vi "ROIAroundGaussian.vi"(9 "Resolution":cluster{"X Step":u16, "Y Step":u16}={"X Step"=1280, "Y Step"=1024}, 10 "Rangefactor (multiple w)":dbl=3.0, 11 "Fit Pixel":dbl[](array[numeric])) -> (0 "Subsampling":i32(ring)=16 items=["1"=1, "2"=2, "4"=4, "8"=8, "16"=16], 1 "ROI Offset":i32[](array[numeric]), 2 "Rectangle":T2 {"Rotation" min=-90.0 max=90.0 step=1.0 format="%.2f"; "Left" scale=0.0..1024.0; "Right" scale=0.0..1024.0}, 3 "ROI":T1, 4 "ROI Width":dbl, 5 "Rectangle (Array)":i32[](array[numeric]))   [LabVIEW 2015]
panel:
  # "x"
  # "pixels"
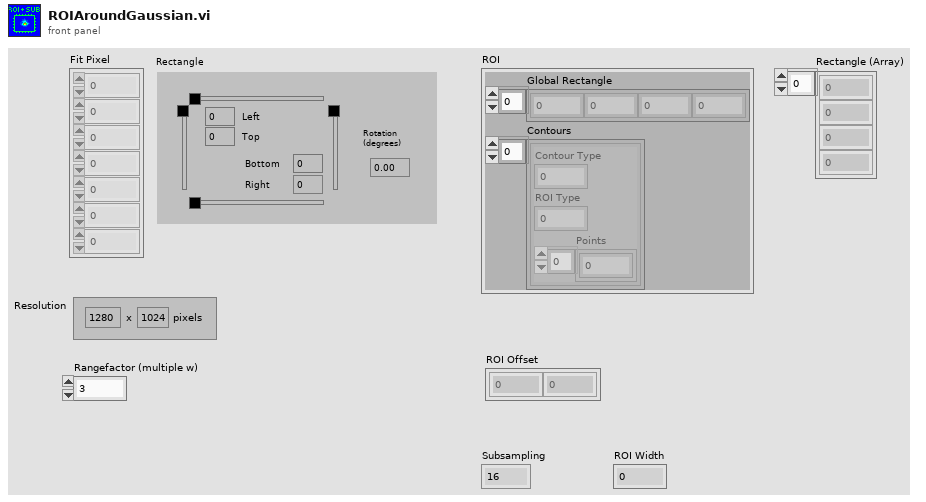
[diagram p1: front panel]
types:
  T1 = cluster{"Global Rectangle":i32[], "Contours":cluster{"Contour Type":u32, "ROI Type":u32, "Points":i32[]}[]}
  T2 = typedef "IMAQ Rectangle" = cluster{"Left":i32, "Top":i32, "Right":i32, "Bottom":i32, "Rotation":dbl}
  T3 = typedef "ROI Descriptor" = cluster{"Global Rectangle":i32[], "Contours":cluster{"ID":enum32{"External", "Internal"}, "Type":u32, "Coordinates":i32[]}[]}
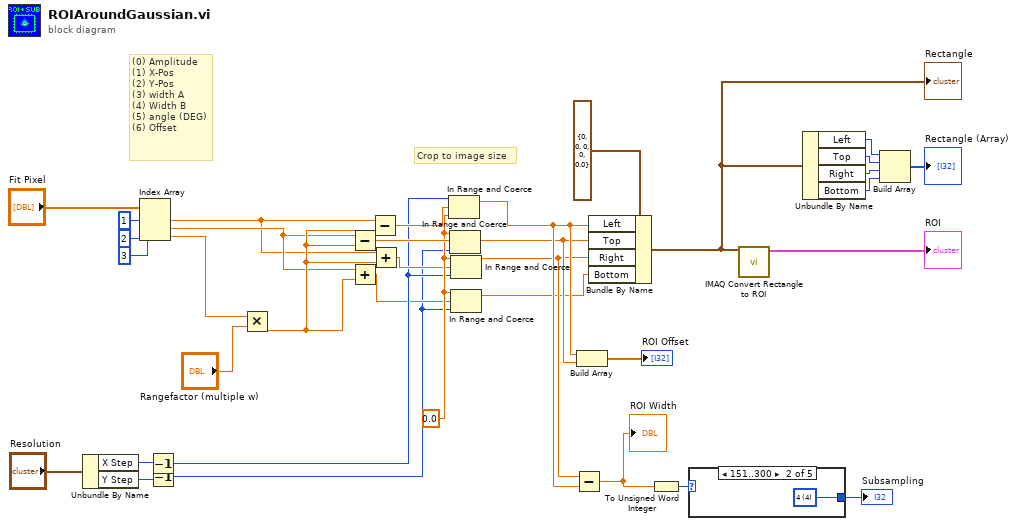
[diagram p0: block diagram]
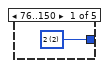
[diagram p2: hidden frame]
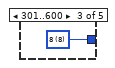
[diagram p3: hidden frame]
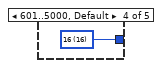
[diagram p4: hidden frame]
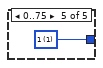
[diagram p5: hidden frame]
diagram:
  w14 = 0.0 ("lower limit")
  # "Crop to image size"
  # "(0) Amplitude\n(1) X-Pos\n(2) Y-Pos\n(3) width A\n(4) Width B\n(5) angle (DEG)\n(6) Offset"
  n1 = Unbundle By Name("Resolution") -> ("X Step"=w20:u16, "Y Step"=w19:u16)
  n2 = Index Array(array="Fit Pixel", index #1=1 ("index"), index #2=2 ("index"), index #3=3 ("index")) -> (element #1=w24:dbl, element #2=w28:dbl, element #3=w31:dbl)
  n3 = Decrement(x=w20) -> (x-1=w11:u16)
  n4 = Decrement(x=w19) -> (x-1=w8:u16)
  n5 = Multiply(x=w31, y="Rangefactor (multiple w)") -> (x*y=w29:dbl)
  n6 = Subtract(x=w28, y=w29) -> (x-y=w16:dbl)
  n7 = Add(x=w28, y=w29) -> (x+y=w10:dbl)
  n8 = Subtract(x=w24, y=w29) -> (x-y=w18:dbl)
  n9 = Add(x=w24, y=w29) -> (x+y=w13:dbl)
  n10 = In Range and Coerce(upper limit=w11, x=w18, lower limit=w14) -> (coerced(x)=w17:dbl)  [unwired: 1 out]
  n11 = In Range and Coerce(upper limit=w14, x=w16, lower limit=w8) -> (coerced(x)=w15:dbl)  [unwired: 1 out]
  n12 = In Range and Coerce(upper limit=w14, x=w13, lower limit=w11) -> (coerced(x)=w12:dbl)  [unwired: 1 out]
  n13 = In Range and Coerce(upper limit=w14, x=w10, lower limit=w8) -> (coerced(x)=w9:dbl)  [unwired: 1 out]
  n14 = Subtract(x=w12, y=w17) -> (x-y=w7:dbl)
  "ROI Width" <- w7
  n15 = Build Array(w17, w15) -> (→"ROI Offset":dbl[])
  n16 = Bundle By Name(cluster=T2 {"Left"=0, "Top"=0, "Right"=0, "Bottom"=0, "Rotation"=0.0} ("Rectangle 2"), "Left"=w17, "Top"=w15, "Right"=w12, "Bottom"=w9) -> (w3:T2)
  "Rectangle" <- w3
  n17 = To Unsigned Word Integer(number=w7) -> (unsigned 16bit integer=w23:u16)
  n18 = case shown="151..300" w23 {
    tunnel: [w36 w37 w38 w39 w40] -> w22
    frame 76..150 {
      w36 = 2 items=["1"=1, "2"=2, "4"=4, "8"=8, "16"=16] ("Subsampling")
    }
    frame 151..300 {
      w37 = 4 items=["1"=1, "2"=2, "4"=4, "8"=8, "16"=16] ("Subsampling")
    }
    frame 301..600 {
      w38 = 8 items=["1"=1, "2"=2, "4"=4, "8"=8, "16"=16] ("Subsampling")
    }
    frame 601..5000, Default {
      w39 = 16 items=["1"=1, "2"=2, "4"=4, "8"=8, "16"=16] ("Subsampling")
    }
    frame 0..75 {
      w40 = 1 items=["1"=1, "2"=2, "4"=4, "8"=8, "16"=16] ("Subsampling")
    }
  }
  "Subsampling" <- w22
  n19 = call "IMAQ Convert Rectangle to ROI"("Rectangle"=w3) -> ("ROI Descriptor"=→"ROI":T3)  [unwired: 8 in, 1 out]
  n20 = Unbundle By Name(w3) -> ("Left"=w1:i32, "Top"=w6:i32, "Right"=w5:i32, "Bottom"=w4:i32)
  n21 = Build Array(w1, w6, w5, w4) -> (→"Rectangle (Array)":i32[])
